vi "main ver.1.0.vi"() -> ()   [LabVIEW 2021]
uses:
  <vilib>/MakerHub/LINX/Public/Peripherals/Digital/Digital Read N Chans.vi
  <vilib>/MakerHub/LINX/Private/Local IO/LinxDigitalRead.vi
  <vilib>/MakerHub/LINX/Public/Utilities/Check Channel.vi
  <vilib>/MakerHub/LINX/Public/Utilities/Open Serial.vi
  <vilib>/MakerHub/LINX/Private/Utilties/Generate Error.vi
  <vilib>/MakerHub/LINX/LMH-LINX.lvlib
panel:
  in  "SAVE":bool
  out "U":string
  out "Values":bool[](array[boolean])
  in  "unit pin":u8[](array[numeric])=[22, 23, 24, 25, 26, 27, 28, 29, 30, 31, 32, 33, 34]
  in  "Value pin":u8[](array[numeric])=[0, 1, 2, 3, 4, 5, 6, 7, 8, 9, 10, 11, 12, 13, 14, 15, 16, 17, 18, 19, 20, 21]
  in  "PATH":path
  in  "STOP":bool
  out "Error Out":errorcluster
  in  "Serial Port":refnum<visa-resource-name>="N/A"
  # "1B\n2B\n11B\n12A\n12B\n10A\n9A\n9B\n10B\n15B\n13A\n13B\n14B\n19B\n17A\n17B\n18B\n23B\n21A\n21B\n22B\n3B"
  # "11A\n16B\n16A\n15A\n14A\n5B\n5A\n6B\n6A\n4A\n7B\n4B\n7A"
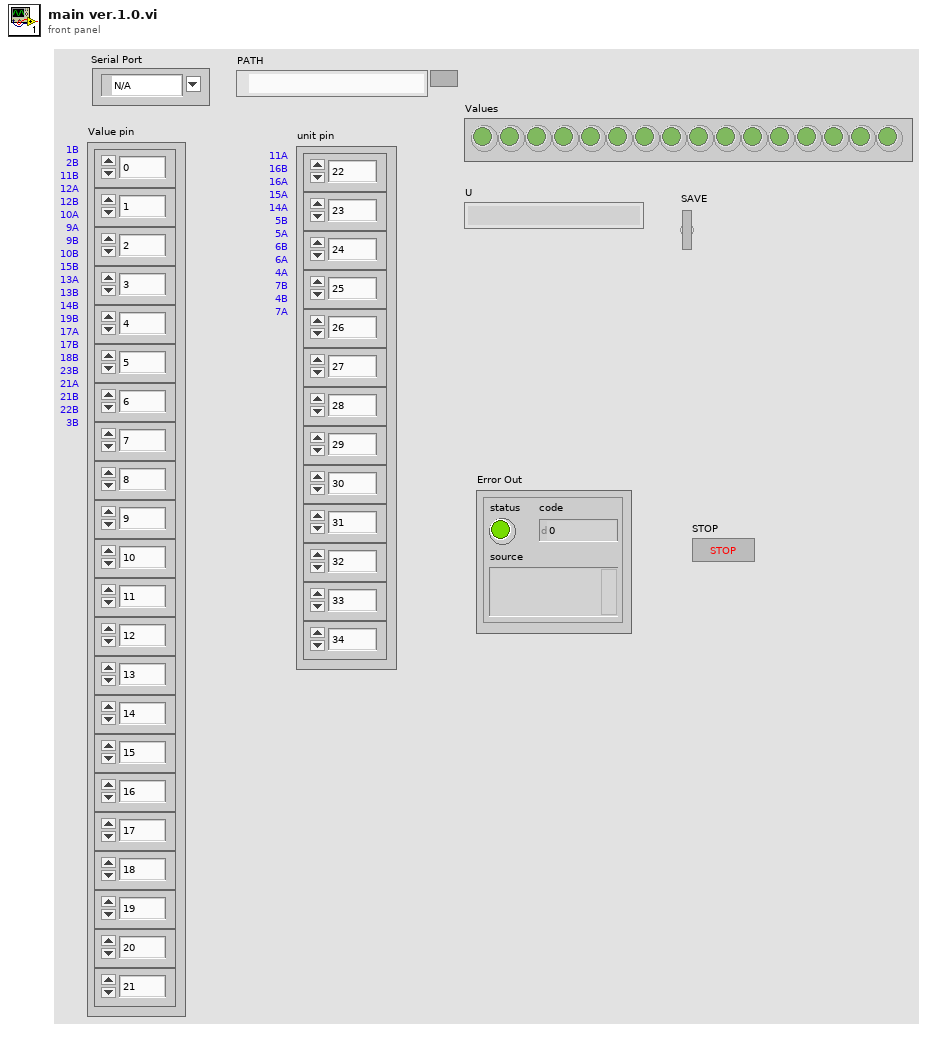
[diagram p1: front panel]
types:
  T1 = typedef "LMH-LINX.lvlib/LINX Ref.ctl" = cluster{"IO":T2, "Interface":T3, "LINX Device Config":T4}
  T2 = typedef "LMH-LINX.lvlib/Platform.ctl" = enum16{"Remote", "Local"}
  T3 = typedef "LMH-LINX.lvlib/Interface.ctl" = enum16{"Serial", "TCP"}
  T4 = typedef "LMH-LINX.lvlib/Device.lvlib/LINX Device Config.ctl" = cluster{"Interface":T3, "COM Port":refnum<visa-resource-name>, "TCP Configuration":T5, "Device Family":u8, "Device ID":u8, "Device Name":string, "TCP Ref":refnum<k5>, "Channels":T6}
  T5 = typedef "LMH-LINX.lvlib/Device.lvlib/TCP Config.ctl" = cluster{"IP Address":string, "Port":u16}
  T6 = typedef "LMH-LINX.lvlib/Channels.ctl" = cluster{"DI":u8[], "DO":u8[], "AI":u8[], "AO":u8[], "PWM":u8[], "QE":u8[], "UART":u8[], "I2C 2":u8[], "SPI":u8[], "CAN":u8[], "Servo":u8[], "AI Ref (V)":dbl, "AI Resolution (Bits)":u8, "AO Ref (V)":dbl, "AO Resolution (Bits)":u8}
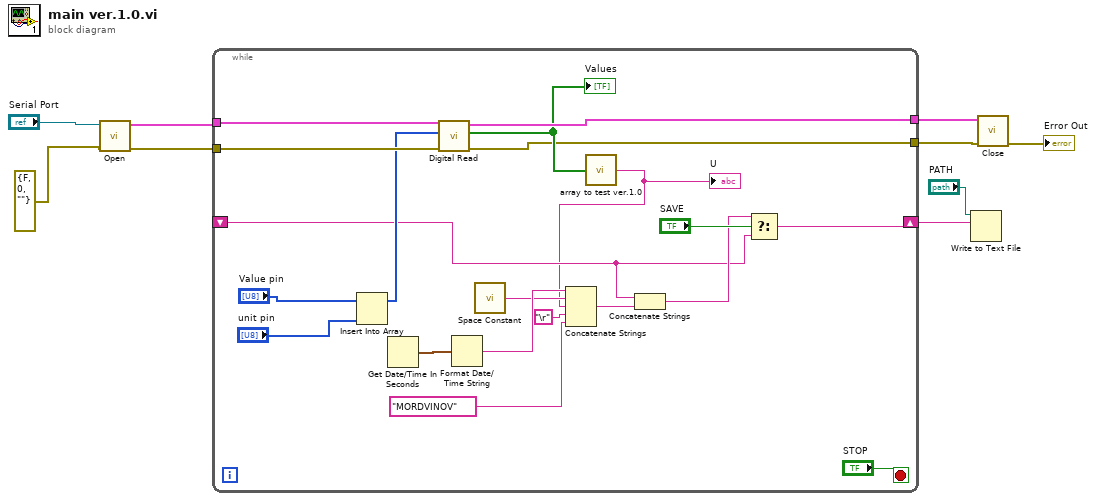
[diagram p0: block diagram]
diagram:
  n1 = call-poly <vilib>:"Open.vi"("Error In"=errorcluster {"status"=FALSE, "code"=0, "source"=""}, "Serial Port"="Serial Port") -> ("Error Out"=w2:errorcluster, "LINX Resource"=w3:T1)  [unwired: 7 in, 1 out]
  n2 = while {
    shift-right: [w14] -> w8
    shift-left: _ -> [w13]
    tunnel: w3 -> [w23]
    tunnel: [w22] -> w6
    tunnel: w2 -> [w21]
    tunnel: [w12] -> w1
    stop <- "STOP" stop-if-true
    n3 = Insert Into Array(array="Value pin", new element="unit pin") -> (w18:u8[])  [unwired: 1 in]
    n4 = Get Date/Time In Seconds() -> (seconds since 1Jan1904=w25:timestamp)
    n5 = call-poly <vilib>:"Digital Read.vi"("Error In"=w21, "DI Channels"=w18, "LINX Resource"=w23) -> ("Error Out"=w12:errorcluster, "Values"=w17:bool[], "LINX Resource"=w22:T1)  [unwired: 6 in]
    "Values" <- w17
    n6 = Format Date/Time String(seconds (now)=w25) -> (date/time string=w28:string)  [unwired: 2 in]
    n7 = call <vilib>:"Space Constant.vi"() -> ("String"=w27:string)
    n8 = call "array to test ver.1.0.vi"("Values"=w17) -> ("output"=w11:string)
    "U" <- w11
    n9 = Concatenate Strings(w28, w27, w11, "\r", "MORDVINOV" ("字符串")) -> (w24:string)
    n10 = Concatenate Strings(w13, w24) -> (w15:string)
    n11 = Select(t=w15, s="SAVE", f=w13) -> (s? t:f=w14:string)
  }
  n12 = Write to Text File(file (use dialog)="PATH", text=w8) -> ()  [unwired: 2 in, 3 out]
  n13 = call <vilib>:"Close.vi"("Error In"=w1, "LINX Resource"=w6) -> ("Error Out"=→"Error Out":errorcluster)  [unwired: 9 in]
